vi "Is Alarm Acknowledged.vi"(11 "Alarm":T1) -> (1 "Alarm Cleared?":bool, 2 "Alarm Set?":bool, 3 "Acknowledged?":bool)   [LabVIEW 2018, in "Dynamic Shared Variables.lvlib"]
uses:
  Dynamic Shared Variables.lvlib
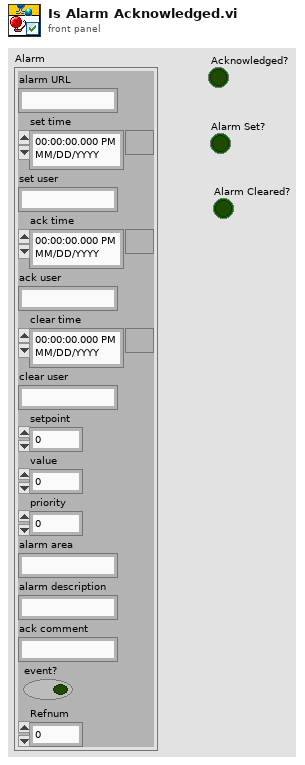
[diagram p1: front panel]
types:
  T1 = cluster{"alarm URL":string, "set time":timestamp, "set user":string, "ack time":timestamp, "ack user":string, "clear time":timestamp, "clear user":string, "setpoint":dbl, "value":dbl, "priority":u32, "alarm area":string, "alarm description":string, "ack comment":string, "event?":bool, "Refnum":u64}
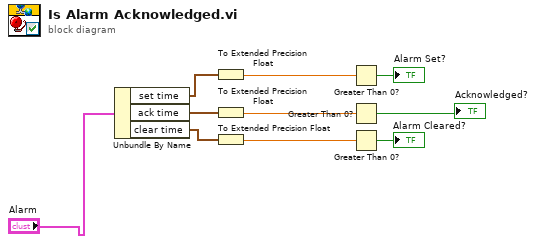
[diagram p0: block diagram]
diagram:
  n1 = Unbundle By Name("Alarm") -> ("set time"=w4:timestamp, "ack time"=w10:timestamp, "clear time"=w3:timestamp)
  n2 = To Extended Precision Float(1:w4) -> (0:w5:ext)
  n3 = To Extended Precision Float(1:w10) -> (0:w7:ext)
  n4 = To Extended Precision Float(1:w3) -> (0:w6:ext)
  n5 = Greater Than 0?(x=w5) -> (x > 0?=→"Alarm Set?":bool)
  n6 = Greater Than 0?(x=w7) -> (x > 0?=→"Acknowledged?":bool)
  n7 = Greater Than 0?(x=w6) -> (x > 0?=→"Alarm Cleared?":bool)
